vi "Output DC Voltage.vi"(0 "COM Port":string="COM3", 1 "Impedance Compensation (0: None)":i32(ring) items=["None", "2-wire", "4-wire"], 2 "+Vmax":dbl=600.0, 3 "+ I Limit":dbl=1.0, 5 "Primary Voltage":dbl, 9 "Output Type":i32(ring) items=["DC Volts", "AC Volts", "DC Current", "AC Current", "DC Power", "AC Power", "Dual DC Volts", "Dual AC Volts", "Resistance"], 11 "error in":errorcluster, 12 "Output Enabled":bool, 13 "-Vmin":dbl=-600.0, 14 "- I Limit":dbl=-5.0) -> (4 "VISA resource name out":refnum<visa-resource-name>="COM3", 15 "error out":errorcluster)   [LabVIEW 2013]
uses:
  <instrlib>/Fluke 5080/Fluke 5080.lvlib
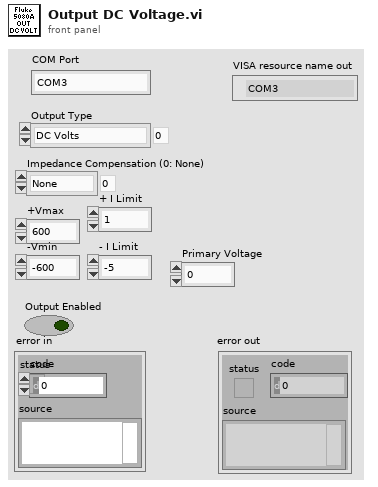
[diagram p1: front panel]
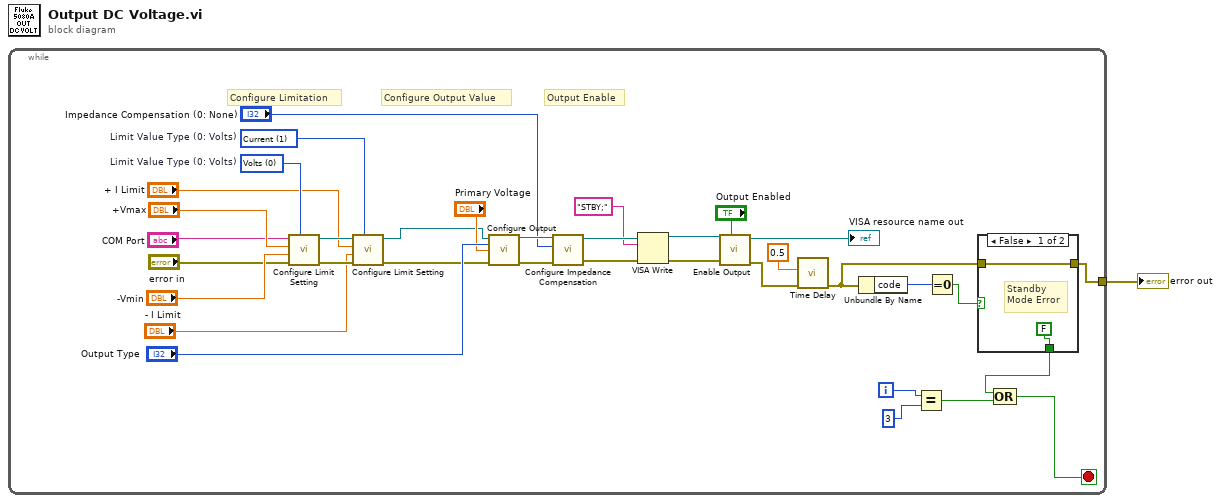
[diagram p0: block diagram]
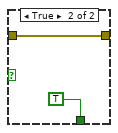
[diagram p2: hidden frame]
diagram:
  n1 = while {
    tunnel: [w2] -> w1
    i -> [w7]
    stop <- w4 stop-if-true
    w28 = 1 items=["Volts", "Current"]  # Limit Value Type (0: Volts)
    w29 = 0 items=["Volts", "Current"]  # Limit Value Type (0: Volts)
    # "Output Enable"
    # "Configure Output Value"
    # "Configure Limitation"
    n2 = call <instrlib>:"Configure Limit Setting.vi"("Limit Value Type (0: Volts)"=w29, "error in (no error)"="error in", "- Limit Value (-5)"="-Vmin", "+ Limit Value (5)"="+Vmax", "VISA resource name"="COM Port") -> ("error out"=w30:errorcluster, "VISA resource name out"=w31:refnum<visa-resource-name>)  [unwired: 5 out]
    n3 = call <instrlib>:"Configure Limit Setting.vi"("Limit Value Type (0: Volts)"=w28, "error in (no error)"=w30, "- Limit Value (-5)"="- I Limit", "+ Limit Value (5)"="+ I Limit", "VISA resource name"=w31) -> ("error out"=w16:errorcluster, "VISA resource name out"=w17:refnum<visa-resource-name>)  [unwired: 5 out]
    n4 = call <instrlib>:"Configure Output.vi"("VISA resource name"=w17, "Output Type (0: DC Volts)"="Output Type", "Primary Voltage (5.0)"="Primary Voltage", "error in (no error)"=w16) -> ("VISA resource name out"=w35:refnum<visa-resource-name>, "error out"=w34:errorcluster)  [unwired: 6 in, 4 out]
    n5 = call <instrlib>:"Configure Impedance Compensation.vi"("error in (no error)"=w34, "Impedance Compensation (0: None)"="Impedance Compensation (0: None)", "VISA resource name"=w35) -> ("error out"=w15:errorcluster, "VISA resource name out"=w14:refnum<visa-resource-name>)  [unwired: 7 out]
    n6 = VISA Write(VISA resource name=w14, write buffer="STBY;", error in (no error)=w15) -> (VISA resource name out=w13:refnum<visa-resource-name>, error out=w12:errorcluster)  [unwired: 1 out]
    n7 = call <instrlib>:"Enable Output.vi"("Output Enabled (T: Enable)"="Output Enabled", "error in (no error)"=w12, "VISA resource name"=w13) -> ("error out"=w20:errorcluster, "VISA resource name out"=→"VISA resource name out":refnum<visa-resource-name>)  [unwired: 7 out]
    n8 = call "Time Delay"("error in (no error)"=w20, "Delay Time (s)"=0.5) -> ("error out"=w3:errorcluster)  [unwired: 9 in]
    n9 = Unbundle By Name(w3) -> ("code"=w10:i32)
    n10 = Equal?(x=w7, y=3) -> (x = y?=w5:bool)
    n11 = Equal To 0?(x=w10) -> (x = 0?=w9:bool)
    n12 = case shown="False" w9 {
      tunnel: [FALSE TRUE] -> w6
      tunnel: w3 -> [w37 w39]
      tunnel: [w37 w39] -> w2
      frame False {
        # "Standby\nMode Error"
      }
      frame True {
      }
    }
    n13 = Compound Arithmetic op=OR(w6, w5) -> (w4:bool)
  }
  "error out" <- w1
